vi "KE2260B Operation Status.vi"(8 "error in (no error)":errorcluster, 11 "VISA resource name":refnum<visa-resource-name>) -> (0 "error out":errorcluster, 1 "CC":bool, 2 "CV":bool, 3 "VISA resource name out":refnum<visa-resource-name>, 4 "Output OFF Delay":bool, 5 "Output ON Delay":bool)   [LabVIEW 2021, in "Keithley 2260B.lvlib"]
doc: "Returns operation status. constant voltage (CV) ,constant current (CC) , output on delay , and output off delay."
uses:
  Keithley 2260B.lvlib
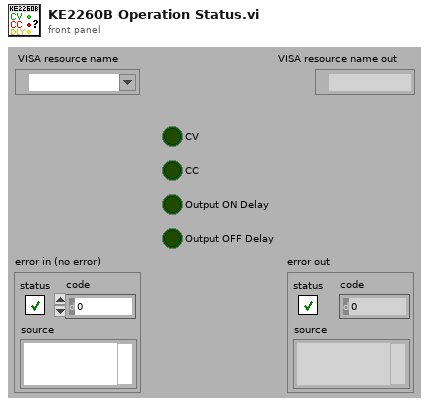
[diagram p1: front panel]
types:
  T1 = cluster{"Boolean array[0]":bool, "Boolean array[1]":bool, "Boolean array[2]":bool, "Boolean array[3]":bool, "Boolean array[4]":bool, "Boolean array[5]":bool, "Boolean array[6]":bool, "Boolean array[7]":bool, "Boolean array[8]":bool, "Boolean array[9]":bool, "Boolean array[10]":bool, "Boolean array[11]":bool, "Boolean array[12]":bool, "Boolean array[13]":bool, "Boolean array[14]":bool, "Boolean array[15]":bool}
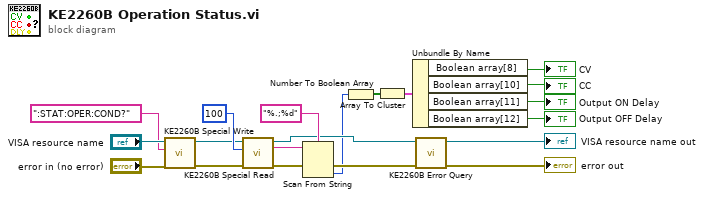
[diagram p0: block diagram]
diagram:
  n1 = call "KE2260B Special Write.vi"("error in (no error)"="error in (no error)", "Write Buffer (\"\")"=":STAT:OPER:COND?" ("write buffer"), "VISA session"="VISA resource name") -> ("error out"=w12:errorcluster, "dup VISA session"=w8:refnum<visa-resource-name>)  [unwired: 6 in, 1 out]
  n2 = call "KE2260B Special Read.vi"("error in (no error)"=w12, "byte count"=u32 100, "VISA session"=w8) -> ("error out"=w15:errorcluster, "read buffer"=w17:string, "dup VISA session"=w13:refnum<visa-resource-name>)  [unwired: 5 in, 1 out]
  n3 = Scan From String(format string="%.;%d", input string=w17, error in=w15) -> (error out=w14:errorcluster, output 1=w5:i32)  [unwired: 2 in, 2 out]
  n4 = Number To Boolean Array(number=w5) -> (Boolean array=w7:bool[])
  n5 = Array To Cluster(array=w7) -> (cluster=w6:T1)
  n6 = Unbundle By Name(w6) -> ("Boolean array[8]"=→"CV":bool, "Boolean array[10]"=→"CC":bool, "Boolean array[11]"=→"Output ON Delay":bool, "Boolean array[12]"=→"Output OFF Delay":bool)
  n7 = call "KE2260B Error Query.vi"("error in (no error)"=w14, "VISA resource name"=w13) -> ("error out"=→"error out":errorcluster, "VISA resource name out"=→"VISA resource name out":refnum<visa-resource-name>)  [unwired: 6 in, 2 out]
